vi "Player Info.vi"(11 "Lone Wolf in":refnum<class "Lone Wolf.lvclass">) -> (1 "Victory Speech":string, 2 "Name":string, 3 "Lone Wolf out":refnum<class "Lone Wolf.lvclass">)   [LabVIEW 2015, in "Lone Wolf.lvclass"]
uses:
  Lone Wolf.lvclass
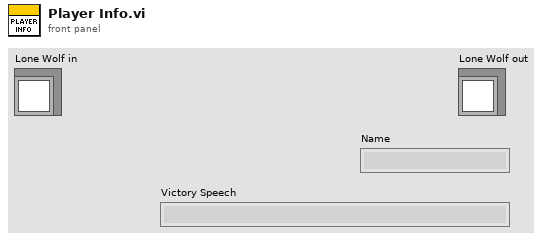
[diagram p1: front panel]
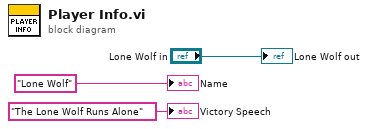
[diagram p0: block diagram]
diagram:
  "Lone Wolf out" <- "Lone Wolf in"
  "Name" <- "Lone Wolf" ("Name")
  "Victory Speech" <- "The Lone Wolf Runs Alone" ("Victory Speech")
